vi "quicktest.vi"() -> ()   [LabVIEW 2009]
panel:
  in  "disable all":bool
  in  "IPR":bool
  out "number 3":u32
  in  "Channel":i32
  out "number 2":u32
  in  "VC_EN":bool=TRUE
  in  "VC_3NS":bool
  in  "VC_2NS":bool
  in  "VC_L":bool
  in  "VC_H":bool
  in  "VC 0.25ns":bool
  out "number":u32
  out "LS_L":string
  out "LS_H":string
  in  "LS_H":i32=72
  in  "reg":i32=18
  out "x/y":dbl
  in  "L1 value":i32=255
  in  "Boolean":bool=TRUE
  in  "vatt":i32=4095
  out "error out":errorcluster
  in  "Vclip":i32
  out "DAC0 Value":i32
  in  "stop":bool
  out "IPR value":i32
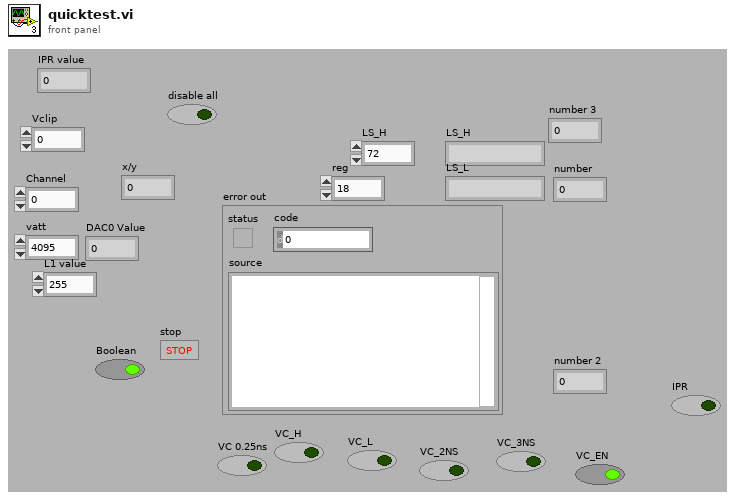
[diagram p1: front panel]
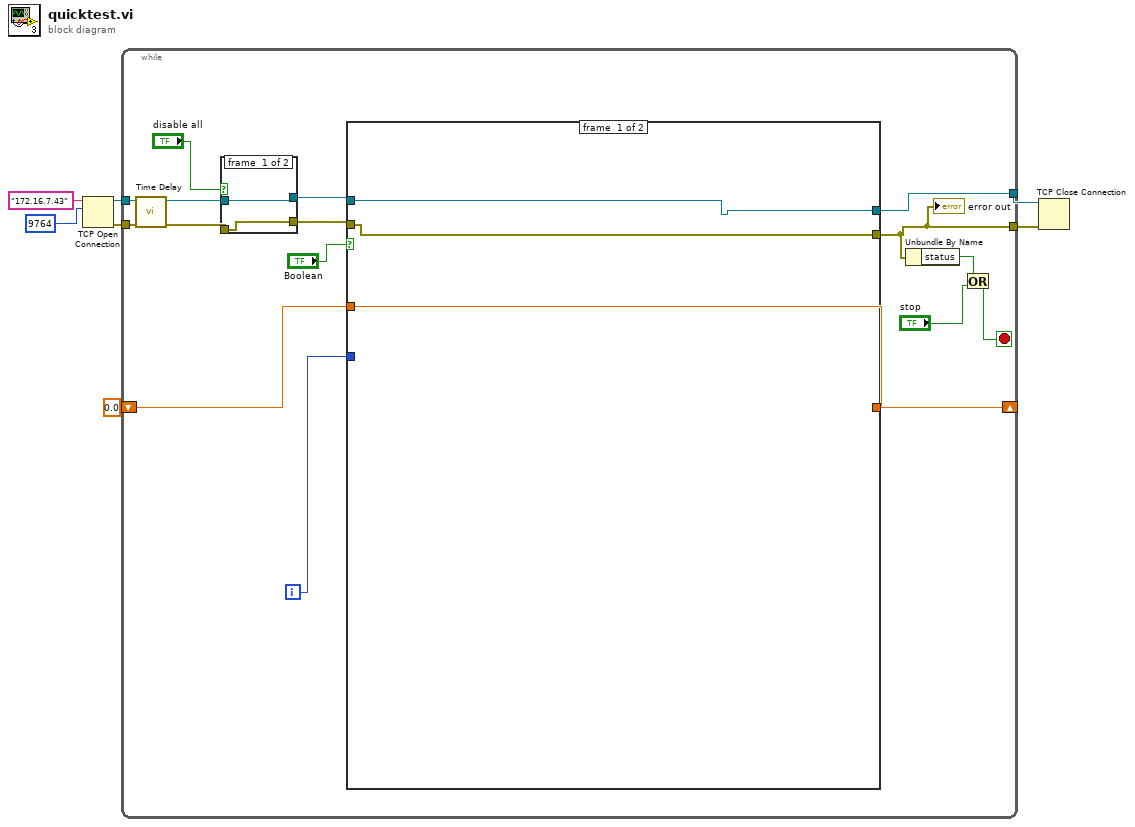
[diagram p0: block diagram]
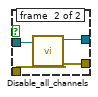
[diagram p2: hidden frame]
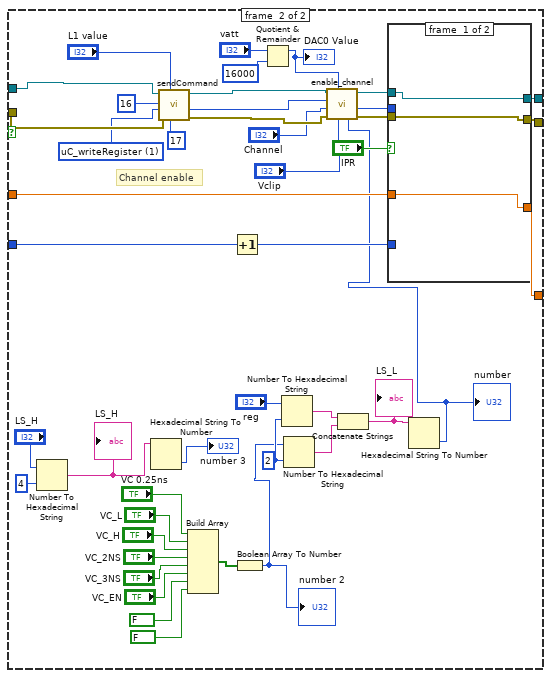
[diagram p3: hidden frame]
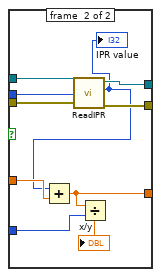
[diagram p4: hidden frame]
diagram:
  n1 = TCP Open Connection(address="172.16.7.43", remote port or service name=u16 9764) -> (connection ID=w7:refnum<k5>, error out=w4:errorcluster)  [unwired: 3 in]
  n2 = while {
    tunnel: w7 -> [w11]
    tunnel: w4 -> [w9]
    tunnel: [w20] -> w3
    tunnel: [w21] -> w2
    shift-right: [w16] -> _
    shift-left: 0.0 -> [w15]
    i -> [w14]
    stop <- w19 stop-if-true
    n3 = call "Time Delay"("error in (no error)"=w9) -> ("error out"=w10:errorcluster)  [unwired: 10 in]
    n4 = case shown="True" "disable all" {
      tunnel: [w23 w28] -> w13
      tunnel: [w24 w27] -> w12
      tunnel: w11 -> [w24 w26]
      tunnel: w10 -> [w23 w25]
      frame #0 {
      }
      frame #1 {
        n5 = call "Disable_all_channels.vi"("error in"=w25, "connection ID"=w26) -> ("error out"=w28:errorcluster, "connection ID out"=w27:refnum<k5>)  [unwired: 7 in, 1 out]
      }
    }
    n6 = case shown="True" "Boolean" {
      tunnel: [w30 w65] -> w20
      tunnel: w13 -> [w30 w50]
      tunnel: w12 -> [w31 w49]
      tunnel: [w31 w64] -> w21
      tunnel: [w29 w51] -> w16
      tunnel: w15 -> [w29 w63]
      tunnel: w14 -> [_ w75]
      frame #0 {
      }
      frame #1 {
        w46 = u16 1 items=["sendCommand"=9, "FPGA_writeRegister"=3, "FPGA_readRegister"=2, "uC_writeRegister"=1, "uC_readRegister"=0] ("Action")
        w66 = i16 2 ("width (-)")
        # "Channel enable"
        n7 = Number To Hexadecimal String(1:i16 4 ("width (-)"), 2:"LS_H") -> (0:w70:string)
        "LS_H" <- w70
        n8 = Hexadecimal String To Number(string=w70) -> (number=→"number 3":u32)  [unwired: 2 in, 1 out]
        n9 = call "sendCommand.vi"("Address"=17, "Data"="L1 value", "error in"=w50, "Action"=w46, "id_in"=16 ("id"), "connection ID"=w49) -> ("error out"=w41:errorcluster, "id_out"=w39:i32, "connection ID out"=w42:refnum<k5>)  [unwired: 1 in, 2 out]
        n10 = Build Array("VC 0.25ns", "VC_L", "VC_H", "VC_2NS", "VC_3NS", "VC_EN", FALSE ("element"), FALSE ("element")) -> (w54:bool[])
        n11 = Increment(x=w75) -> (x+1=w74:i32)
        n12 = Boolean Array To Number(Boolean array=w54) -> (number=w53:u32)
        "number 2" <- w53
        n13 = Quotient & Remainder(x="vatt", y=16000) -> (x-y*floor(x/y)=w37:i32)  [unwired: 1 out]
        "DAC0 Value" <- w37
        n14 = Number To Hexadecimal String(1:w66, 2:"reg") -> (0:w68:string)
        n15 = Number To Hexadecimal String(1:w66, 2:w53) -> (0:w69:string)
        n16 = Concatenate Strings(w68, w69) -> (w73:string)
        "LS_L" <- w73
        n17 = Hexadecimal String To Number(string=w73) -> (number=w32:u32)  [unwired: 2 in, 1 out]
        "number" <- w32
        n18 = call "enable_channel.vi"("Delay"=w32, "V clip"="Vclip", "V att"=w37, "error in"=w41, "Channel"="Channel", "id_in"=w39, "connection ID"=w42) -> ("error out"=w40:errorcluster, "id_out"=w38:i32, "connection ID out"=w43:refnum<k5>)  [unwired: 2 in]
        n19 = case shown="True" "IPR" {
          tunnel: w74 -> [_ w88]
          tunnel: [w77 w87] -> w65
          tunnel: [w76 w86] -> w64
          tunnel: w63 -> [w78 w85]
          tunnel: [w78 w82] -> w51
          tunnel: w43 -> [w76 w81]
          tunnel: w40 -> [w77 w80]
          tunnel: w38 -> [_ w79]
          frame #0 {
          }
          frame #1 {
            n20 = call "ReadIPR.vi"("error in"=w80, "id_in"=w79, "connection ID"=w81) -> ("error out"=w87:errorcluster, "IPR value"=w84:i32, "connection ID out"=w86:refnum<k5>)  [unwired: 6 in]
            "IPR value" <- w84
            n21 = Add(x=w84, y=w85) -> (x+y=w82:dbl)
            n22 = Divide(x=w82, y=w88) -> (x/y=→"x/y":dbl)
          }
        }
      }
    }
    "error out" <- w20
    n23 = Unbundle By Name(w20) -> ("status"=w18:bool)
    n24 = Or(x=w18, y="stop") -> (x .or. y?=w19:bool)
  }
  n25 = TCP Close Connection(connection ID=w2, error in (no error)=w3) -> ()  [unwired: 1 in, 2 out]
